vi "SUB_Parsing_from_table_to_cluster.vi"(11 "ROM Table":string[][](table)=[["Device ID", "303012001", "-"], ["YEAR", "16", "-"], ["Month", "11", "-"], ["Day", "09", "-"], ["Device Type(HEX)", "1F42", "-"], ["Manufacturer ID", "14872", "-"], ["Cal_Scale A (HEX)", "44", "-"], ["Cal_Scale B (HEX)", "43", "-"], ["Cal_Acc. X", "29116", "-"], ["Cal_Acc. Y", "29682", "-"], ["Cal_Acc. Z", "32727", "-"], ["Cal_Gy. X", "41378", "-"], ["Cal_Gy. Y", "45490", "-"], ["Cal_Gy. Z", "49602", "-"], ["Cal_Vol H", "44850", "-"], ["Cal_Vol L", "34000", "-"], ["Cal_CDC Off 1", "4370", "-"], ["Cal_CDC Off 2", "8482", "-"], ["Cal_CDC Off 3", "12594", "-"], ["Cal_CDC Off 4", "16706", "-"], ["Cal_CDC Off 5", "20818", "-"], ["Cal_CDC Off 6", "24930", "-"], ["Cal_CDC Off 7", "29042", ""], ["Cal_CDC Off 8", "33154", ""]]) -> (1 "PCAP zero information":T2 {"Sensor 8" format="%x"; "Sensor 7" format="%x"; "Sensor 6" format="%x"; "Sensor 5" format="%x"; "Sensor 4" format="%x"; "Sensor 3" format="%x"; "Sensor 2" format="%x"; "Sensor 1" format="%x"; "Packet ID" format="%x"}, 2 "Cal information":T3 {"Voltage L 2.8V" format="%x"; "Voltage H 2.8V" format="%x"; "Voltage L 3.1V" format="%x"; "Acc Z_L_Cal" format="%x"; "Voltage H 3.1V" format="%x"; "Gyro Z_L_Cal" format="%x"; "Gyro Z_H_Cal" format="%x"; "Gyro Y_L_Cal" format="%x"; "Gyro Y_H_Cal" format="%x"; "Gyro X_L_Cal" format="%x"; "Gyro X_H_Cal" format="%x"; "Acc Z_H_Cal" format="%x"; "Acc Y_L_Cal" format="%x"; "Acc Y_H_Cal" format="%x"; "Acc X_L_Cal" format="%x"; "Acc X_H_Cal" format="%x"; "Packet ID" format="%x"}, 3 "Device information":T1 {"Device Type L" format="%x"; "Device Type H" format="%x"; "Check sum" format="%x"; "Scale B" format="%x"; "Scale A" format="%x"; "Manufacturer Lot ID 4" format="%x"; "Manufacturer Lot ID 3" format="%x"; "Manufacturer Lot ID 2" format="%x"; "Manufacturer Lot ID 1" format="%x"; "Day" format="%x"; "Month" format="%x"; "Year" format="%x"; "Device ID 4" format="%x"; "Device ID 3" format="%x"; "Device ID 2" format="%x"; "Device ID 1" format="%x"; "Packet ID" format="%x"})   [LabVIEW 2015]
uses:
  Cluster Type/Cal information.ctl
  Cluster Type/PCAP zero information.ctl
  Cluster Type/Device information.ctl
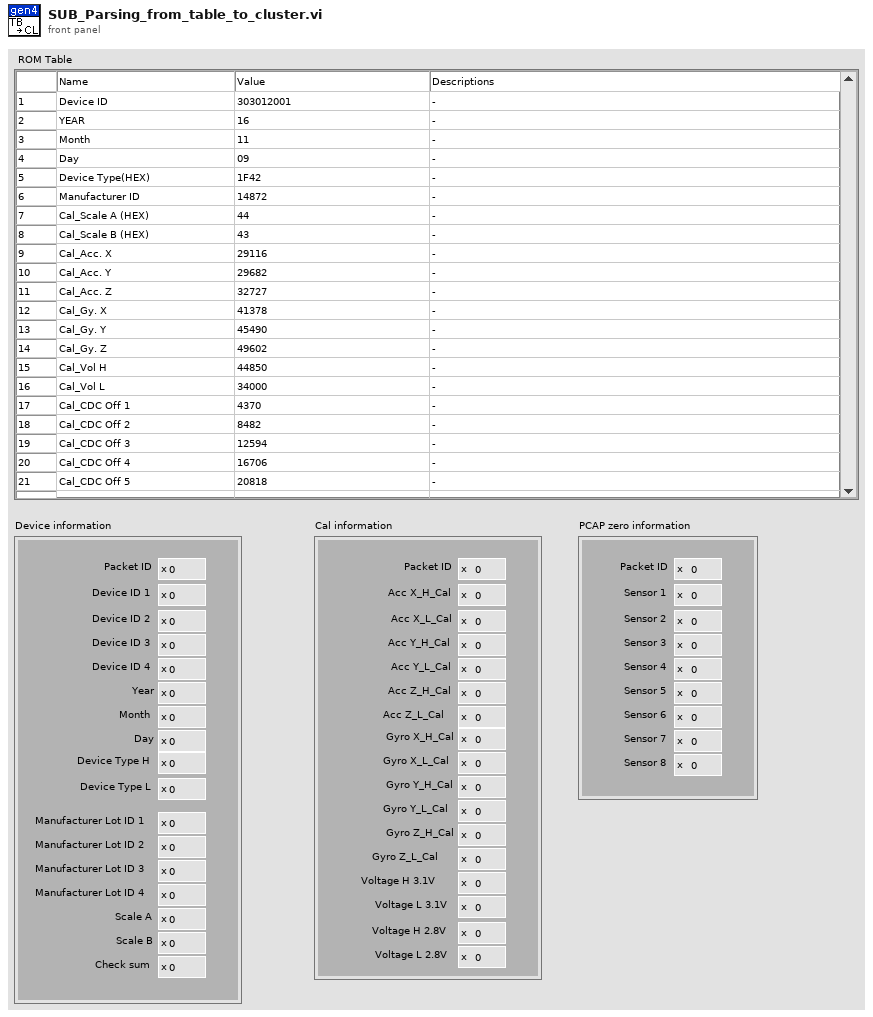
[diagram p1: front panel]
types:
  T1 = typedef "Device information.ctl" = cluster{"Packet ID":u8, "Device ID 1":u8, "Device ID 2":u8, "Device ID 3":u8, "Device ID 4":u8, "Year":u8, "Month":u8, "Day":u8, "Device Type H":u8, "Device Type L":u8, "Manufacturer Lot ID 1":u8, "Manufacturer Lot ID 2":u8, "Manufacturer Lot ID 3":u8, "Manufacturer Lot ID 4":u8, "Scale A":u8, "Scale B":u8, "Check sum":u8}
  T2 = typedef "PCAP zero information.ctl" = cluster{"Packet ID":u8, "Sensor 1":u16, "Sensor 2":u16, "Sensor 3":u16, "Sensor 4":u16, "Sensor 5":u16, "Sensor 6":u16, "Sensor 7":u16, "Sensor 8":u16}
  T3 = typedef "Cal information.ctl" = cluster{"Packet ID":u8, "Acc X_H_Cal":u8, "Acc X_L_Cal":u8, "Acc Y_H_Cal":u8, "Acc Y_L_Cal":u8, "Acc Z_H_Cal":u8, "Acc Z_L_Cal":u8, "Gyro X_H_Cal":u8, "Gyro X_L_Cal":u8, "Gyro Y_H_Cal":u8, "Gyro Y_L_Cal":u8, "Gyro Z_H_Cal":u8, "Gyro Z_L_Cal":u8, "Voltage H 3.1V":u8, "Voltage L 3.1V":u8, "Voltage H 2.8V":u8, "Voltage L 2.8V":u8}
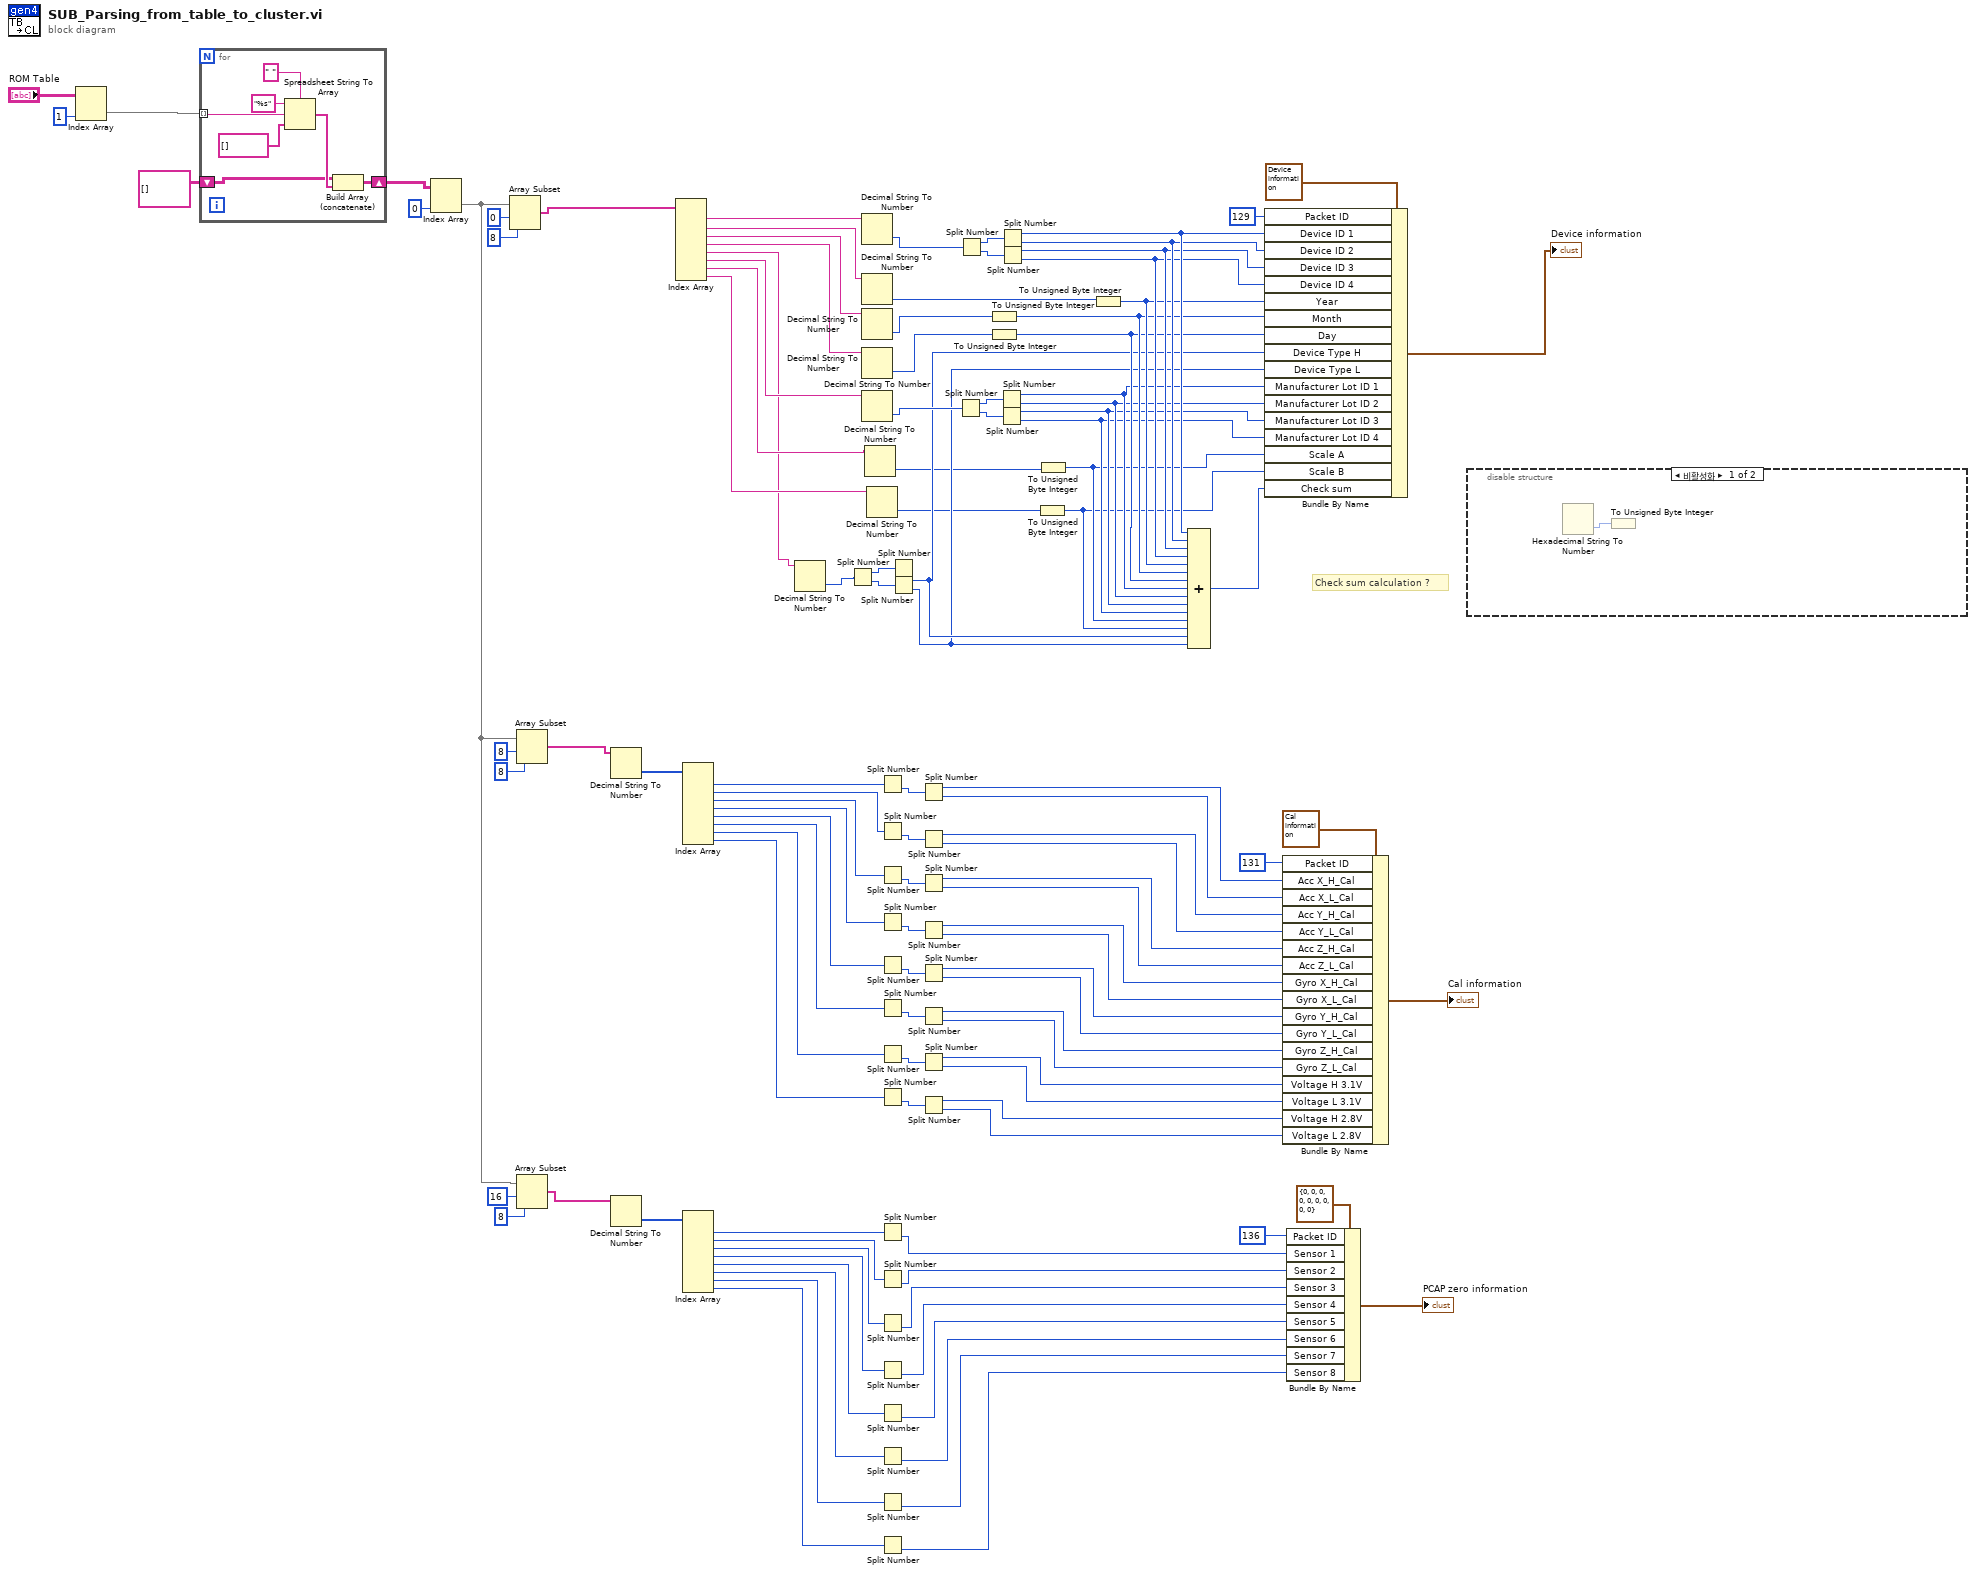
[diagram p0: block diagram]
diagram:
  # "Check sum calculation ?"
  n1 = Index Array(array="ROM Table", index (col)=1 ("비활성화된 인덱스 (열)")) -> (element=w12:string[])  [unwired: 1 in]
  n2 = for {
    tunnel: w12 -> [w120] mode=indexing
    shift-right: [w115] -> w9
    shift-left: string[][] [] -> [w114]
    n3 = Spreadsheet String To Array(delimiter (Tab)=" " ("구분 문자(탭)"), format string="%s" ("포맷 문자열"), spreadsheet string=w120, array type (2D Dbl)=string[] []) -> (array=w116:string[])
    n4 = Build Array (concatenate)(w114, w116) -> (w115:string[][])
  }
  n5 = Index Array(array=w9, index (col)=0 ("비활성화된 인덱스 (열)")) -> (element=w8:string[])  [unwired: 1 in]
  n6 = Array Subset(array=w8, index=0 ("인덱스"), length=8 ("길이")) -> (w75:string[])
  n7 = Array Subset(array=w8, index=8 ("인덱스"), length=8 ("길이")) -> (w70:string[])
  n8 = Array Subset(array=w8, index=16 ("인덱스"), length=8 ("길이")) -> (w30:string[])
  n9 = Decimal String To Number(string=w70) -> (number=w69:i32[])  [unwired: 2 in, 1 out]
  n10 = Decimal String To Number(string=w30) -> (number=w31:i32[])  [unwired: 2 in, 1 out]
  n11 = Index Array(array=w75) -> (element #1=w90:string, element #2=w88:string, element #3=w87:string, element #4=w86:string, element #5=w2:string, element #6=w83:string, element #7=w6:string, element #8=w5:string)  [unwired: 8 in]
  n12 = Index Array(array=w69) -> (element #1=w68:i32, element #2=w60:i32, element #3=w59:i32, element #4=w56:i32, element #5=w55:i32, element #6=w54:i32, element #7=w53:i32, element #8=w52:i32)  [unwired: 8 in]
  n13 = Index Array(array=w31) -> (element #1=w29:i32, element #2=w27:i32, element #3=w26:i32, element #4=w25:i32, element #5=w24:i32, element #6=w23:i32, element #7=w22:i32, element #8=w21:i32)  [unwired: 8 in]
  n14 = Decimal String To Number(string=w2) -> (number=w1:i32)  [unwired: 2 in, 1 out]
  n15 = Split Number(x=w1) -> (hi(x)=w81:u16, lo(x)=w80:u16)
  n16 = Decimal String To Number(string=w90) -> (number=w89:i32)  [unwired: 2 in, 1 out]
  n17 = Decimal String To Number(string=w88) -> (number=w7:i32)  [unwired: 2 in, 1 out]
  n18 = Decimal String To Number(string=w87) -> (number=w85:i32)  [unwired: 2 in, 1 out]
  n19 = Decimal String To Number(string=w86) -> (number=w84:i32)  [unwired: 2 in, 1 out]
  n20 = Decimal String To Number(string=w83) -> (number=w82:i32)  [unwired: 2 in, 1 out]
  n21 = Decimal String To Number(string=w6) -> (number=w4:i32)  [unwired: 2 in, 1 out]
  n22 = Decimal String To Number(string=w5) -> (number=w3:i32)  [unwired: 2 in, 1 out]
  n23 = Split Number(x=w68) -> (lo(x)=w71:u16)  [unwired: 1 out]
  n24 = Split Number(x=w60) -> (lo(x)=w65:u16)  [unwired: 1 out]
  n25 = Split Number(x=w59) -> (lo(x)=w64:u16)  [unwired: 1 out]
  n26 = Split Number(x=w56) -> (lo(x)=w63:u16)  [unwired: 1 out]
  n27 = Split Number(x=w55) -> (lo(x)=w62:u16)  [unwired: 1 out]
  n28 = Split Number(x=w54) -> (lo(x)=w61:u16)  [unwired: 1 out]
  n29 = Split Number(x=w53) -> (lo(x)=w57:u16)  [unwired: 1 out]
  n30 = Split Number(x=w52) -> (lo(x)=w58:u16)  [unwired: 1 out]
  n31 = Split Number(x=w29) -> (lo(x)=w28:u16)  [unwired: 1 out]
  n32 = Split Number(x=w27) -> (lo(x)=w20:u16)  [unwired: 1 out]
  n33 = Split Number(x=w26) -> (lo(x)=w19:u16)  [unwired: 1 out]
  n34 = Split Number(x=w25) -> (lo(x)=w18:u16)  [unwired: 1 out]
  n35 = Split Number(x=w24) -> (lo(x)=w17:u16)  [unwired: 1 out]
  n36 = Split Number(x=w23) -> (lo(x)=w16:u16)  [unwired: 1 out]
  n37 = Split Number(x=w22) -> (lo(x)=w14:u16)  [unwired: 1 out]
  n38 = Split Number(x=w21) -> (lo(x)=w15:u16)  [unwired: 1 out]
  n39 = Split Number(x=w81) -> ()  [unwired: 2 out]
  n40 = Split Number(x=w80) -> (hi(x)=w79:u8, lo(x)=w78:u8)
  n41 = Split Number(x=w71) -> (hi(x)=w67:u8, lo(x)=w66:u8)
  n42 = Split Number(x=w65) -> (hi(x)=w51:u8, lo(x)=w50:u8)
  n43 = Split Number(x=w64) -> (hi(x)=w49:u8, lo(x)=w48:u8)
  n44 = Split Number(x=w63) -> (hi(x)=w47:u8, lo(x)=w46:u8)
  n45 = Split Number(x=w62) -> (hi(x)=w45:u8, lo(x)=w44:u8)
  n46 = Split Number(x=w61) -> (hi(x)=w43:u8, lo(x)=w42:u8)
  n47 = Split Number(x=w57) -> (hi(x)=w41:u8, lo(x)=w40:u8)
  n48 = Split Number(x=w58) -> (hi(x)=w39:u8, lo(x)=w38:u8)
  n49 = Split Number(x=w82) -> (hi(x)=w106:u16, lo(x)=w107:u16)
  n50 = Split Number(x=w89) -> (hi(x)=w112:u16, lo(x)=w111:u16)
  n51 = To Unsigned Byte Integer(number=w85) -> (unsigned 8bit integer=w99:u8)
  n52 = To Unsigned Byte Integer(number=w84) -> (unsigned 8bit integer=w98:u8)
  n53 = Split Number(x=w106) -> (hi(x)=w97:u8, lo(x)=w96:u8)
  n54 = Split Number(x=w107) -> (hi(x)=w95:u8, lo(x)=w94:u8)
  n55 = Split Number(x=w112) -> (hi(x)=w104:u8, lo(x)=w103:u8)
  n56 = Split Number(x=w111) -> (hi(x)=w102:u8, lo(x)=w101:u8)
  n57 = To Unsigned Byte Integer(number=w3) -> (unsigned 8bit integer=w92:u8)
  n58 = To Unsigned Byte Integer(number=w4) -> (unsigned 8bit integer=w93:u8)
  n59 = To Unsigned Byte Integer(number=w7) -> (unsigned 8bit integer=w100:u8)
  n60 = Compound Arithmetic op=ADD(w104, w103, w102, w101, w100, w99, w98, w97, w96, w95, w94, w93, w92, w79, w78) -> (w105:u8)
  n61 = Bundle By Name(cluster=T1 {"Packet ID"=0, "Device ID 1"=0, "Device ID 2"=0, "Device ID 3"=0, "Device ID 4"=0, "Year"=0, "Month"=0, "Day"=0, "Device Type H"=0, "Device Type L"=0, "Manufacturer Lot ID 1"=0, "Manufacturer Lot ID 2"=0, "Manufacturer Lot ID 3"=0, "Manufacturer Lot ID 4"=0, "Scale A"=0, "Scale B"=0, "Check sum"=0} ("Device information"), "Packet ID"=u8 129, "Device ID 1"=w104, "Device ID 2"=w103, "Device ID 3"=w102, "Device ID 4"=w101, "Year"=w100, "Month"=w99, "Day"=w98, "Device Type H"=w79, "Device Type L"=w78, "Manufacturer Lot ID 1"=w97, "Manufacturer Lot ID 2"=w96, "Manufacturer Lot ID 3"=w95, "Manufacturer Lot ID 4"=w94, "Scale A"=w93, "Scale B"=w92, "Check sum"=w105) -> (→"Device information":T1)
  n62 = Bundle By Name(cluster=T3 {"Packet ID"=0, "Acc X_H_Cal"=0, "Acc X_L_Cal"=0, "Acc Y_H_Cal"=0, "Acc Y_L_Cal"=0, "Acc Z_H_Cal"=0, "Acc Z_L_Cal"=0, "Gyro X_H_Cal"=0, "Gyro X_L_Cal"=0, "Gyro Y_H_Cal"=0, "Gyro Y_L_Cal"=0, "Gyro Z_H_Cal"=0, "Gyro Z_L_Cal"=0, "Voltage H 3.1V"=0, "Voltage L 3.1V"=0, "Voltage H 2.8V"=0, "Voltage L 2.8V"=0} ("Cal information"), "Packet ID"=u8 131, "Acc X_H_Cal"=w67, "Acc X_L_Cal"=w66, "Acc Y_H_Cal"=w51, "Acc Y_L_Cal"=w50, "Acc Z_H_Cal"=w49, "Acc Z_L_Cal"=w48, "Gyro X_H_Cal"=w47, "Gyro X_L_Cal"=w46, "Gyro Y_H_Cal"=w45, "Gyro Y_L_Cal"=w44, "Gyro Z_H_Cal"=w43, "Gyro Z_L_Cal"=w42, "Voltage H 3.1V"=w41, "Voltage L 3.1V"=w40, "Voltage H 2.8V"=w39, "Voltage L 2.8V"=w38) -> (→"Cal information":T3)
  n63 = Bundle By Name(cluster=T2 {"Packet ID"=0, "Sensor 1"=0, "Sensor 2"=0, "Sensor 3"=0, "Sensor 4"=0, "Sensor 5"=0, "Sensor 6"=0, "Sensor 7"=0, "Sensor 8"=0} ("PCAP zero information"), "Packet ID"=u8 136, "Sensor 1"=w28, "Sensor 2"=w20, "Sensor 3"=w19, "Sensor 4"=w18, "Sensor 5"=w17, "Sensor 6"=w16, "Sensor 7"=w14, "Sensor 8"=w15) -> (→"PCAP zero information":T2)
  n64 = disable-structure shown="비활성화" {
    frame Disabled {
      n65 = Hexadecimal String To Number() -> (number=w121:u32)  [unwired: 3 in, 1 out]
      n66 = To Unsigned Byte Integer(number=w121) -> ()  [unwired: 1 out]
    }
    frame Enabled {
    }
  }
